vi "NI VeriStand - Add Child Nodes.vi"(8 "Error in":errorcluster, 10 "Child Nodes":u64[](array[numeric]), 11 "Runtime Configuration Ref in":refnum<k24>) -> (0 "Error out":errorcluster, 1 "Child Nodes":refnum<k24>[](array[refnum]), 2 "Success":bool, 3 "Runtime Configuration Ref out":refnum<k24>)   [LabVIEW 2025, in "NI_VS RuntimeConfigurationFile ScriptingAPI.lvlib"]
uses:
  NI_VS RuntimeConfigurationFile ScriptingAPI.lvlib
  NationalInstruments.VeriStand.SystemDefinitionAPI
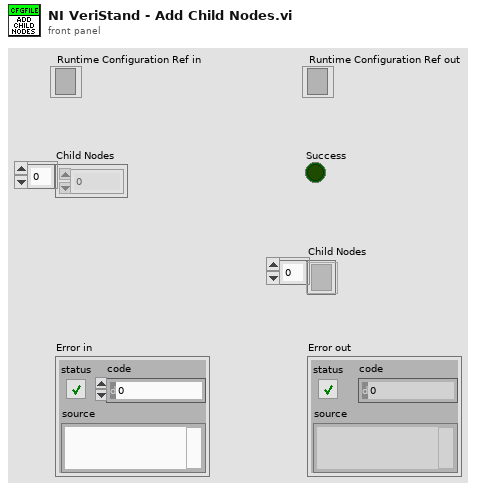
[diagram p1: front panel]
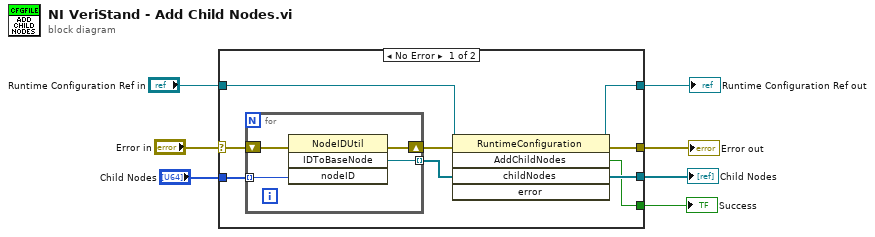
[diagram p0: block diagram]
diagram:
  n1 = case shown="No Error" "Error in" {
    selector: "Error in" -> [w15 _]
    tunnel: "Runtime Configuration Ref in" -> [w13 w21]
    tunnel: [w12 w21] -> w4
    tunnel: [w11 _] -> w3
    tunnel: [w16 _] -> w7
    tunnel: "Child Nodes" -> [w10 _]
    tunnel: [w8 _] -> w1
    frame No Error {
      n2 = for {
        tunnel: w10 -> [w18] mode=indexing
        shift-right: [w19] -> w14
        shift-left: w15 -> [w20]
        tunnel: [w17] -> w9 mode=indexing
        n3 = invoke class="NodeIDUtil" method="IDToBaseNode"(error in=w20, "nodeID"=w18) -> (error out=w19:errorcluster, "IDToBaseNode"=w17:refnum<k24>)  [unwired: 2 in, 2 out]
      }
      n4 = invoke class="RuntimeConfiguration" method="AddChildNodes"(reference=w13, error in=w14, "childNodes"=w9) -> (reference out=w12:refnum<k24>, error out=w16:errorcluster, "AddChildNodes"=w8:bool, "childNodes"=w11:refnum<k24>[])  [unwired: 2 in, 1 out]
    }
    frame Error {
    }
  }
  "Runtime Configuration Ref out" <- w4
  "Success" <- w1
  "Child Nodes" <- w3
  "Error out" <- w7
